vi "Piecewise linear function.vi"() -> ()   [LabVIEW 2020]
panel:
  in  "Image Path":path
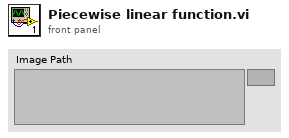
[diagram p1: front panel]
types:
  T1 = typedef "IMAQ Image.ctl" = refnum<image>
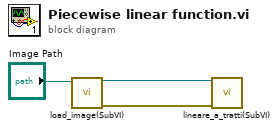
[diagram p0: block diagram]
diagram:
  n1 = call "load_image(SubVI).vi"("Image Path"="Image Path") -> ("error out"=w2:errorcluster, "Image GRAY"=w3:T1)  [unwired: 9 in]
  n2 = call "lineare_a_tratti(SubVI).vi"("image in"=w3, "error in (no error)"=w2) -> ()  [unwired: 10 in, 4 out]
